vi "Main 2.1.vi"() -> ()   [LabVIEW 2022 SP3]
uses:
  <vilib>/MakerHub/LINX/Public/Utilities/Open Serial.vi
  <vilib>/MakerHub/LINX/Public/Sensors/Motion/Servo/Servo Open One Channel.vi
  Global 2 Horizontal.vi
  Global 3 Vertical.vi
  Global 4 Gripper.vi
  Global 1 Base.vi
  <vilib>/MakerHub/LINX/Public/Sensors/Motion/Servo/Servo Set Pulse Width One Channel.vi
  <vilib>/MakerHub/LINX/Public/Sensors/Motion/Servo/Servo Close One Channel.vi
  Global 5 grid number.vi
  Global 6 Bool.vi
  <vilib>/MakerHub/LINX/LMH-LINX.lvlib
  <vilib>/MakerHub/LINX/Public/Sensors/Motion/Servo/Servo.lvlib
panel:
  out "Square 2":dynamicdata(graph) caption="Square"
  out "Object detected":bool=TRUE
  out "Object not detected / Unreachable":bool=TRUE
  out "Base":i32
  out "Gripper":i32
  out "Vertical":i32
  out "Horzontal":i32
  out "Grid No":i32
  out "Starting":bool=TRUE
  out "Waiting":bool
  out "Over":bool=TRUE
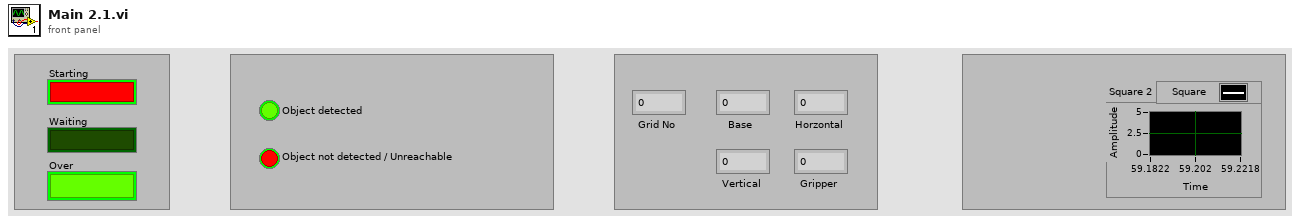
[diagram p1: front panel]
types:
  T1 = typedef "LMH-LINX.lvlib/LINX Ref.ctl" = cluster{"IO":T2, "Interface":T3, "LINX Device Config":T4}
  T2 = typedef "LMH-LINX.lvlib/Platform.ctl" = enum16{"Remote", "Local"}
  T3 = typedef "LMH-LINX.lvlib/Interface.ctl" = enum16{"Serial", "TCP"}
  T4 = typedef "LMH-LINX.lvlib/Device.lvlib/LINX Device Config.ctl" = cluster{"Interface":T3, "COM Port":refnum<visa-resource-name>, "TCP Configuration":T5, "Device Family":u8, "Device ID":u8, "Device Name":string, "TCP Ref":refnum<k5>, "Channels":T6}
  T5 = typedef "LMH-LINX.lvlib/Device.lvlib/TCP Config.ctl" = cluster{"IP Address":string, "Port":u16}
  T6 = typedef "LMH-LINX.lvlib/Channels.ctl" = cluster{"DI":u8[], "DO":u8[], "AI":u8[], "AO":u8[], "PWM":u8[], "QE":u8[], "UART":u8[], "I2C 2":u8[], "SPI":u8[], "CAN":u8[], "Servo":u8[], "AI Ref (V)":dbl, "AI Resolution (Bits)":u8, "AO Ref (V)":dbl, "AO Resolution (Bits)":u8}
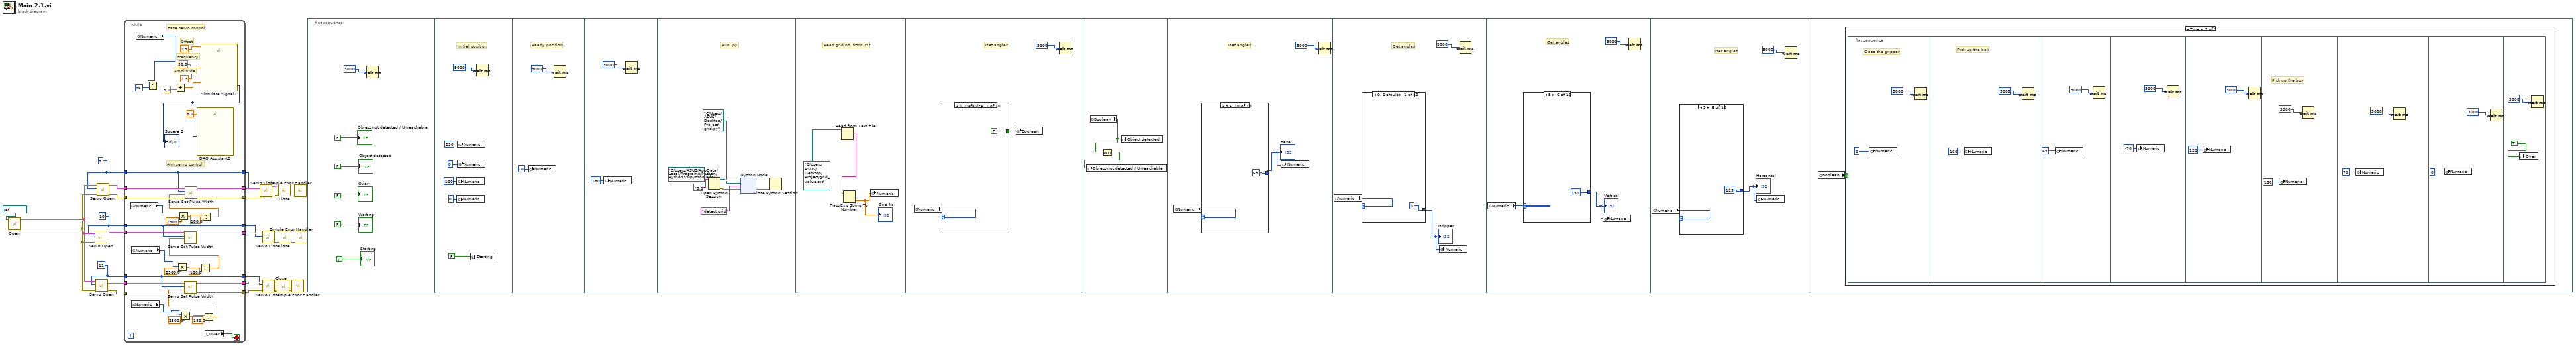
[diagram p0: block diagram]
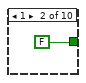
[diagram p2: hidden frame]
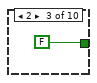
[diagram p3: hidden frame]
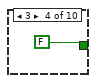
[diagram p4: hidden frame]
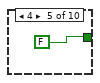
[diagram p5: hidden frame]
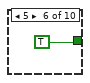
[diagram p6: hidden frame]
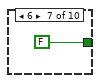
[diagram p7: hidden frame]
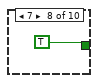
[diagram p8: hidden frame]
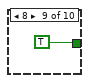
[diagram p9: hidden frame]
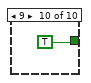
[diagram p10: hidden frame]
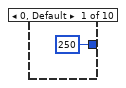
[diagram p11: hidden frame]
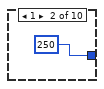
[diagram p12: hidden frame]
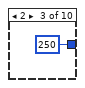
[diagram p13: hidden frame]
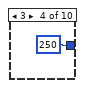
[diagram p14: hidden frame]
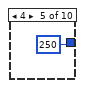
[diagram p15: hidden frame]
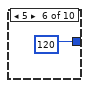
[diagram p16: hidden frame]
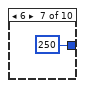
[diagram p17: hidden frame]
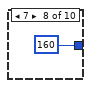
[diagram p18: hidden frame]
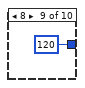
[diagram p19: hidden frame]
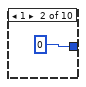
[diagram p20: hidden frame]
diagram:
  w6 = 11
  w4 = 10
  w1 = 9
  n1 = call-poly <vilib>:"Open.vi"("Serial Port"=refnum<visa-resource-name> "COM6") -> ("Error Out"=w7:errorcluster, "LINX Resource"=w8:T1)  [unwired: 8 in, 1 out]
  n2 = call-poly <vilib>:"Servo Open.vi"("Error In"=w7, "Servo Channel"=w4, "LINX Resource"=w8) -> ("LINX Resource"=w14:T1)  [unwired: 7 in, 1 out]
  n3 = call-poly <vilib>:"Servo Open.vi"("Error In"=w7, "Servo Channel"=w6, "LINX Resource"=w8) -> ("Error Out"=w10:errorcluster, "LINX Resource"=w11:T1)  [unwired: 7 in]
  n4 = call-poly <vilib>:"Servo Open.vi"("Error In"=w7, "Servo Channel"=w1, "LINX Resource"=w8) -> ("Error Out"=w25:errorcluster, "LINX Resource"=w27:T1)  [unwired: 7 in]
  n5 = while {
    tunnel: w27 -> [w67]
    tunnel: [w66] -> w26
    tunnel: w25 -> [w65]
    tunnel: [w64] -> w24
    tunnel: w1 -> [w55]
    tunnel: w14 -> [w63]
    tunnel: [w62] -> w13
    tunnel: [w61] -> w12
    tunnel: w11 -> [w60]
    tunnel: w10 -> [w59]
    tunnel: [w58] -> w9
    tunnel: w6 -> [w57]
    tunnel: [w57] -> w5
    tunnel: w4 -> [w56]
    tunnel: [w56] -> w3
    tunnel: [w55] -> w2
    stop <- w29 stop-if-true
    # "Arm servo control"
    # "Base servo control"
    # "Amplitude"
    # "Frequency"
    # "Offset"
    n6 = global read "Global 2 Horizontal.vi" "Numeric"() -> (w40:i32)
    n7 = global read "Global 4 Gripper.vi" "Numeric"() -> (w42:i32)
    n8 = global read "Global 3 Vertical.vi" "Numeric"() -> (w41:i32)
    n9 = global read "Global 1 Base.vi" "Numeric"() -> (w30:i32)
    n10 = Divide(x=w30, y=36) -> (x/y=w32:dbl)
    n11 = Add(x=w32, y=5.0) -> (x+y=w33:dbl)
    n12 = Multiply(x=w41, y=2500.0) -> (x*y=w51:dbl)
    n13 = Multiply(x=w40, y=2500.0) -> (x*y=w54:dbl)
    n14 = Multiply(x=w42, y=2500.0) -> (x*y=w48:dbl)
    n15 = Divide(x=w51, y=180.0) -> (x/y=w44:dbl)
    n16 = call-poly <vilib>:"Servo Set Pulse Width.vi"("Pulse Width (uS)"=w44, "Servo Channel"=w56, "LINX Resource"=w63) -> ("LINX Resource"=w62:T1)  [unwired: 7 in, 1 out]
    n17 = Divide(x=w54, y=180.0) -> (x/y=w43:dbl)
    n18 = call-poly <vilib>:"Servo Set Pulse Width.vi"("Error In"=w65, "Pulse Width (uS)"=w43, "Servo Channel"=w55, "LINX Resource"=w67) -> ("Error Out"=w64:errorcluster, "LINX Resource"=w66:T1)  [unwired: 6 in]
    n19 = call "Simulate Signal2"("Offset"=2.5, "Duty Cycle (%)"=w33, "Frequency"=50.0, "Amplitude"=2.5) -> ("Square"=w39:dynamicdata)  [unwired: 10 in, 1 out]
    "Square 2" <- w39
    n20 = call "DAQ Assistant2"("data"=w39, "timeout (s)"=5.0) -> ()  [unwired: 15 in, 3 out]
    n21 = Divide(x=w48, y=180.0) -> (x/y=w45:dbl)
    n22 = call-poly <vilib>:"Servo Set Pulse Width.vi"("Error In"=w59, "Pulse Width (uS)"=w45, "Servo Channel"=w57, "LINX Resource"=w60) -> ("Error Out"=w58:errorcluster, "LINX Resource"=w61:T1)  [unwired: 6 in]
    n23 = local read "Over"() -> (w29:bool)
  }
  n24 = call-poly <vilib>:"Servo Close.vi"("Error In"=w24, "Servo Channel"=w2, "LINX Resource"=w26) -> ("Error Out"=w21:errorcluster, "LINX Resource"=w22:T1)  [unwired: 7 in]
  n25 = call-poly <vilib>:"Servo Close.vi"("Servo Channel"=w3, "LINX Resource"=w13) -> ("Error Out"=w18:errorcluster, "LINX Resource"=w19:T1)  [unwired: 8 in]
  n26 = call-poly <vilib>:"Servo Close.vi"("Error In"=w9, "Servo Channel"=w5, "LINX Resource"=w12) -> ("Error Out"=w15:errorcluster, "LINX Resource"=w16:T1)  [unwired: 7 in]
  n27 = call <vilib>:"Close.vi"("Error In"=w15, "LINX Resource"=w16) -> ("Error Out"=w17:errorcluster)  [unwired: 9 in]
  n28 = call <vilib>:"Close.vi"("Error In"=w21, "LINX Resource"=w22) -> ("Error Out"=w23:errorcluster)  [unwired: 9 in]
  n29 = call <vilib>:"Close.vi"("Error In"=w18, "LINX Resource"=w19) -> ("Error Out"=w20:errorcluster)  [unwired: 9 in]
  n30 = call <vilib>:"Simple Error Handler.vi"("error in (no error)"=w17) -> ()  [unwired: 4 in, 5 out]
  n31 = call <vilib>:"Simple Error Handler.vi"("error in (no error)"=w23) -> ()  [unwired: 4 in, 5 out]
  n32 = call <vilib>:"Simple Error Handler.vi"("error in (no error)"=w20) -> ()  [unwired: 4 in, 5 out]
  n33 = flat-sequence {
    frame #0 {
      n34 = Wait (ms)(milliseconds to wait=u32 3000 ("millisecond timer value")) -> ()  [unwired: 1 out]
      "Object not detected / Unreachable" <- FALSE
      "Object detected" <- FALSE
      "Over" <- FALSE
      "Waiting" <- FALSE
      "Starting" <- TRUE
    }
    frame #1 {
      # "Initial position"
      n35 = global write "Global 3 Vertical.vi" "Numeric"(160 ("Numeric")) -> ()
      n36 = global write "Global 4 Gripper.vi" "Numeric"(0 ("Numeric")) -> ()
      n37 = global write "Global 1 Base.vi" "Numeric"(250 ("Numeric")) -> ()
      n38 = global write "Global 2 Horizontal.vi" "Numeric"(0 ("Numeric")) -> ()
      n39 = local write "Starting"(FALSE) -> ()
      n40 = Wait (ms)(milliseconds to wait=u32 5000 ("millisecond timer value")) -> ()  [unwired: 1 out]
    }
    frame #2 {
      # "Ready position"
      n41 = global write "Global 2 Horizontal.vi" "Numeric"(70 ("Numeric")) -> ()
      n42 = Wait (ms)(milliseconds to wait=u32 3000 ("millisecond timer value")) -> ()  [unwired: 1 out]
    }
    frame #3 {
      n43 = global write "Global 3 Vertical.vi" "Numeric"(180 ("Numeric")) -> ()
      n44 = Wait (ms)(milliseconds to wait=u32 3000 ("millisecond timer value")) -> ()  [unwired: 1 out]
    }
    frame #4 {
      # "Run .py"
      n45 = Open Python Session(python version="3.9" ("Python version"), python path=path "C:/Users/ASUS/AppData/Local/Programs/Python/Python39/python.exe" ("Python path")) -> (session out=w86:refnum<k35>, error out=w85:errorcluster)  [unwired: 1 in]
      n46 = node "Python Node"(w86, path "C:/Users/ASUS/Desktop/Project/grid.py" ("module path"), "detect_grid" ("function name"), w85) -> (w89:refnum<k35>, w88:errorcluster)  [unwired: 2 in, 2 out]
      n47 = Close Python Session(session in=w89, error in=w88) -> ()  [unwired: 1 out]
    }
    frame #5 {
      # "Read grid no. from .txt"
      n48 = Read from Text File(file (use dialog)=path "C:/Users/ASUS/Desktop/Project/grid_value.txt") -> (text=w93:string)  [unwired: 3 in, 3 out]
      n49 = Fract/Exp String To Number(string=w93) -> (number=w92:dbl)  [unwired: 3 in, 1 out]
      "Grid No" <- w92
      n50 = global write "Global 5 grid number.vi" "Numeric"(w92) -> ()
    }
    frame #6 {
      # "Get angles"
      n51 = global read "Global 5 grid number.vi" "Numeric"() -> (w97:i32)
      n52 = case shown="0, Default" w97 {
        tunnel: [FALSE FALSE FALSE FALSE FALSE TRUE FALSE TRUE TRUE TRUE] -> w96
        frame 0, Default {
        }
        frame 1 {
        }
        frame 2 {
        }
        frame 3 {
        }
        frame 4 {
        }
        frame 5 {
        }
        frame 6 {
        }
        frame 7 {
        }
        frame 8 {
        }
        frame 9 {
        }
      }
      n53 = global write "Global 6 Bool.vi" "Boolean"(w96) -> ()
      n54 = Wait (ms)(milliseconds to wait=u32 3000 ("millisecond timer value")) -> ()  [unwired: 1 out]
    }
    frame #7 {
      n55 = global read "Global 6 Bool.vi" "Boolean"() -> (w109:bool)
      n56 = Not(x=w109) -> (.not. x?=w108:bool)
      n57 = local write "Object not detected / Unreachable"(w108) -> ()
      n58 = local write "Object detected"(w109) -> ()
    }
    frame #8 {
      # "Get angles"
      n59 = global read "Global 5 grid number.vi" "Numeric"() -> (w112:i32)
      n60 = case shown="9" w112 {
        tunnel: [250 250 250 250 250 120 250 160 120 65] -> w111
        frame 0, Default {
        }
        frame 1 {
        }
        frame 2 {
        }
        frame 3 {
        }
        frame 4 {
        }
        frame 5 {
        }
        frame 6 {
        }
        frame 7 {
        }
        frame 8 {
        }
        frame 9 {
        }
      }
      "Base" <- w111
      n61 = global write "Global 1 Base.vi" "Numeric"(w111) -> ()
      n62 = Wait (ms)(milliseconds to wait=u32 3000 ("millisecond timer value")) -> ()  [unwired: 1 out]
    }
    frame #9 {
      # "Get angles"
      n63 = global read "Global 5 grid number.vi" "Numeric"() -> (w124:i32)
      n64 = case shown="0, Default" w124 {
        tunnel: [0 0 0 0 0 130 0 130 130 130] -> w125
        frame 0, Default {
        }
        frame 1 {
        }
        frame 2 {
        }
        frame 3 {
        }
        frame 4 {
        }
        frame 5 {
        }
        frame 6 {
        }
        frame 7 {
        }
        frame 8 {
        }
        frame 9 {
        }
      }
      "Gripper" <- w125
      n65 = global write "Global 4 Gripper.vi" "Numeric"(w125) -> ()
      n66 = Wait (ms)(milliseconds to wait=u32 3000 ("millisecond timer value")) -> ()  [unwired: 1 out]
    }
    frame #10 {
      # "Get angles"
      n67 = global read "Global 5 grid number.vi" "Numeric"() -> (w138:i32)
      n68 = case shown="5" w138 {
        tunnel: [160 160 160 160 160 150 160 150 140 153] -> w137
        frame 0, Default {
        }
        frame 1 {
        }
        frame 2 {
        }
        frame 3 {
        }
        frame 4 {
        }
        frame 5 {
        }
        frame 6 {
        }
        frame 7 {
        }
        frame 8 {
        }
        frame 9 {
        }
      }
      "Vertical" <- w137
      n69 = global write "Global 3 Vertical.vi" "Numeric"(w137) -> ()
      n70 = Wait (ms)(milliseconds to wait=u32 3000 ("millisecond timer value")) -> ()  [unwired: 1 out]
    }
    frame #11 {
      # "Get angles"
      n71 = global read "Global 5 grid number.vi" "Numeric"() -> (w150:i32)
      n72 = case shown="5" w150 {
        tunnel: [60 60 60 60 60 115 60 108 105 105] -> w151
        frame 0, Default {
        }
        frame 1 {
        }
        frame 2 {
        }
        frame 3 {
        }
        frame 4 {
        }
        frame 5 {
        }
        frame 6 {
        }
        frame 7 {
        }
        frame 8 {
        }
        frame 9 {
        }
      }
      "Horzontal" <- w151
      n73 = global write "Global 2 Horizontal.vi" "Numeric"(w151) -> ()
      n74 = Wait (ms)(milliseconds to wait=u32 3000 ("millisecond timer value")) -> ()  [unwired: 1 out]
    }
    frame #12 {
      n75 = global read "Global 6 Bool.vi" "Boolean"() -> (w162:bool)
      n76 = case shown="True" w162 {
        frame False {
          n77 = flat-sequence {
            frame #0 {
              n78 = global read "Global 6 Bool.vi" "Boolean"() -> (w163:bool)
              n79 = local write "Object not detected / Unreachable"(w163) -> ()
            }
            frame #1 {
              n80 = local write "Waiting"(TRUE) -> ()
              n81 = Wait (ms)(milliseconds to wait=u32 10000) -> ()  [unwired: 1 out]
            }
            frame #2 {
              n82 = local write "Waiting"(FALSE) -> ()
              n83 = Wait (ms)(milliseconds to wait=u32 3000) -> ()  [unwired: 1 out]
              n84 = local write "Over"(TRUE) -> ()
            }
          }
        }
        frame True {
          n85 = flat-sequence {
            frame #0 {
              # "Close the gripper"
              n86 = global write "Global 4 Gripper.vi" "Numeric"(0) -> ()
              n87 = Wait (ms)(milliseconds to wait=u32 3000 ("millisecond timer value")) -> ()  [unwired: 1 out]
            }
            frame #1 {
              # "Pick up the box"
              n88 = global write "Global 3 Vertical.vi" "Numeric"(160) -> ()
              n89 = Wait (ms)(milliseconds to wait=u32 3000 ("millisecond timer value")) -> ()  [unwired: 1 out]
            }
            frame #2 {
              n90 = global write "Global 2 Horizontal.vi" "Numeric"(65) -> ()
              n91 = Wait (ms)(milliseconds to wait=u32 3000 ("millisecond timer value")) -> ()  [unwired: 1 out]
            }
            frame #3 {
              n92 = global write "Global 1 Base.vi" "Numeric"(-70 ("Numeric")) -> ()
              n93 = Wait (ms)(milliseconds to wait=u32 3000 ("millisecond timer value")) -> ()  [unwired: 1 out]
            }
            frame #4 {
              n94 = global write "Global 4 Gripper.vi" "Numeric"(120) -> ()
              n95 = Wait (ms)(milliseconds to wait=u32 3000 ("millisecond timer value")) -> ()  [unwired: 1 out]
            }
            frame #5 {
              # "Pick up the box"
              n96 = global write "Global 3 Vertical.vi" "Numeric"(180) -> ()
              n97 = Wait (ms)(milliseconds to wait=u32 3000 ("millisecond timer value")) -> ()  [unwired: 1 out]
            }
            frame #6 {
              n98 = global write "Global 2 Horizontal.vi" "Numeric"(70) -> ()
              n99 = Wait (ms)(milliseconds to wait=u32 3000 ("millisecond timer value")) -> ()  [unwired: 1 out]
            }
            frame #7 {
              n100 = global write "Global 4 Gripper.vi" "Numeric"(0) -> ()
              n101 = Wait (ms)(milliseconds to wait=u32 3000 ("millisecond timer value")) -> ()  [unwired: 1 out]
            }
            frame #8 {
              n102 = local write "Over"(TRUE) -> ()
              n103 = Wait (ms)(milliseconds to wait=u32 3000 ("millisecond timer value")) -> ()  [unwired: 1 out]
            }
          }
        }
      }
    }
  }
